vi "Status - Querry Carrier.vi"(8 "error in":errorcluster, 11 "Configuration Cluster":T1={"Name"="Default Settings", "IP"="192.168.0.84", "Control Port"=4220, "Timeout (ms)"=2000, "Continuous Capture Port (Multiplexed)"=4210, "Start HIL Shot Port"=53999, "AWG Upload Port (Multiplexed)"=54201, "Download Captured Data Port (Multiplexed)"=53000, "Module Slots"=2, "Module Configurations"=[{"Name"="ACQ 425 ELF", "Position"="192.168.0.84", "Module Type"=enum."Analog In Module", "Control Port"=4221, "Timeout (ms)"=2000, "Channels"=16}, {"Name"="AO 424 ELF", "Position"="192.168.0.84", "Module Type"=enum."Analog Out Module", "Control Port"=4222, "Timeout (ms)"=2000, "Channels"=16}]}) -> (0 "error out":errorcluster, 2 "Module Carrier Status":T4, 5 "Timed Out":bool=TRUE)   [LabVIEW 2017, in "Communications Library.lvlib"]
doc: "Querries the status of the DTACQ device.\n\nThe status of the module carrier."
uses:
  Communications Library.lvlib
  Typedefs/DTACQ Module Carrier Status.ctl
  Typedefs/DTACQ Status--Enum.ctl
  Typedefs/DTACQ Module Carrier Configuration--Cluster.ctl
  Typedefs/DTACQ Module Configuration--Cluster.ctl
  Typedefs/DTACQ Device Type--Enum.ctl
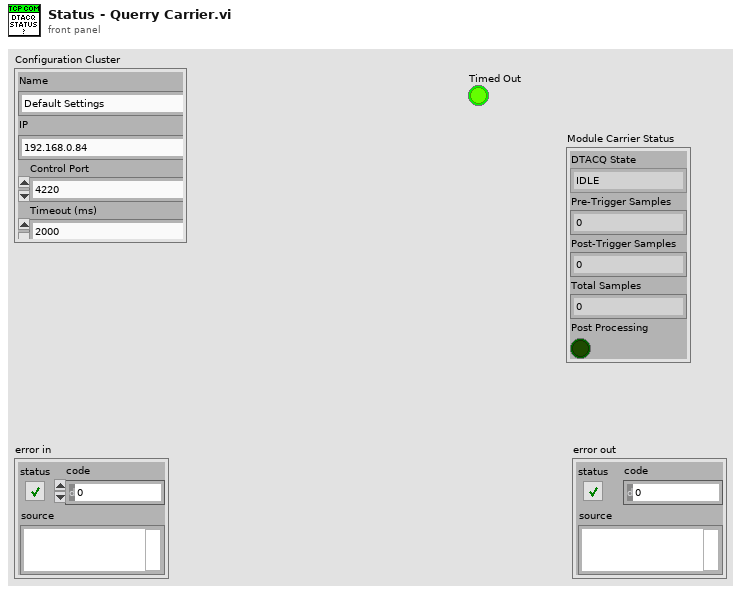
[diagram p1: front panel]
types:
  T1 = typedef "Communications Library.lvlib/DTACQ Module Carrier Configuration--Cluster.ctl" = cluster{"Name":string, "IP":string, "Control Port":i32, "Timeout (ms)":i32, "Continuous Capture Port (Multiplexed)":i32, "Start HIL Shot Port":i32, "AWG Upload Port (Multiplexed)":i32, "Download Captured Data Port (Multiplexed)":i32, "Module Slots":i32, "Module Configurations":T2[]}
  T2 = typedef "Communications Library.lvlib/DTACQ Module Configuration--Cluster.ctl" = cluster{"Name":string, "Position":string, "Module Type":T3, "Control Port":i32, "Timeout (ms)":i32, "Channels":i32}
  T3 = typedef "Communications Library.lvlib/DTACQ Device Type--Enum.ctl" = enum16{"Carrier", "Analog In Module", "Analog Out Module", "Generic Module"}
  T4 = typedef "Communications Library.lvlib/DTACQ Module Carrier Status.ctl" = cluster{"DTACQ State":T5, "Pre-Trigger Samples":i32, "Post-Trigger Samples":i32, "Total Samples":i32, "Post Processing":bool}
  T5 = typedef "Communications Library.lvlib/DTACQ Status--Enum.ctl" = enum16{"IDLE", "ARM", "RUN_PRE-TRIGGER", "RUN_POST-TRIGGER", "POST_PROCESS", "CLEANUP"}
  T6 = typedef "Communications Library.lvlib/DTACQ Connection Data--Cluster.ctl" = cluster{"Description":string, "Address":string, "Port":u16, "timeout (ms)":i32, "Termination Character":string, "TCP Connection Reference":refnum<k5>, "Open Connection":bool}
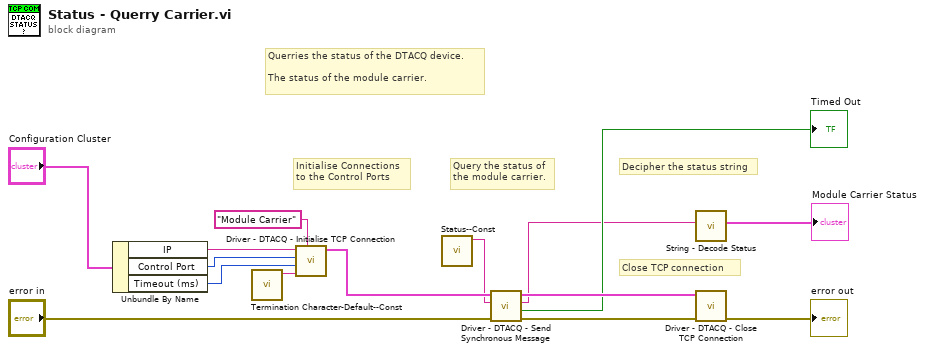
[diagram p0: block diagram]
diagram:
  # "Querries the status of the DTACQ device.\n\nThe status of the module carrier."
  # "Close TCP connection"
  # "Decipher the status string"
  # "Query the status of\nthe module carrier."
  # "Initialise Connections\nto the Control Ports"
  n1 = Unbundle By Name("Configuration Cluster") -> ("IP"=w5:string, "Control Port"=w4:i32, "Timeout (ms)"=w3:i32)
  n2 = call "Termination Character-Default--Const.vi"() -> ("Termination Character"=w14:string)  [unwired: 11 in]
  n3 = call "Driver - DTACQ - Initialise TCP Connection.vi"("Description"="Module Carrier", "Termination Character"=w14, "timeout (ms)"=w3, "Port"=w4, "Address"=w5) -> ("DTACQ Connection Data Out"=w13:T6)  [unwired: 6 in]
  n4 = call "Status--Const.vi"() -> ("Status Command"=w12:string)  [unwired: 11 in]
  n5 = call "Driver - DTACQ - Send Synchronous Message.vi"("error in"="error in", "Message to Send"=w12, "DTACQ Connection Data In"=w13) -> ("error out"=w11:errorcluster, "Timed Out"=→"Timed Out":bool, "Read String"=w7:string, "DTACQ Connection Data Out"=w10:T6)  [unwired: 5 in]
  n6 = call "String - Decode Status.vi"("Status Response String"=w7) -> ("Module Carrier Status"=→"Module Carrier Status":T4)  [unwired: 9 in, 1 out]
  n7 = call "Driver - DTACQ - Close TCP Connection.vi"("error in"=w11, "DTACQ Connection Data In"=w10) -> ("error out"=→"error out":errorcluster)  [unwired: 8 in, 1 out]
